vi "Check_Temps.vi"(8 "error in (no error)":errorcluster, 10 "Temperatures":sgl[][](array[numeric]), 11 "Alarm_Data In":T4) -> (0 "error out":errorcluster, 3 "Alarm_Data out":T4)   [LabVIEW 2019, in "Alarm_Manager.lvlib"]
uses:
  Alarm_Manager.lvlib
  Alarm_Data.ctl
  Message_Handler/typedef/Alarm_Panel.ctl
  Channel_Temperature_Threshold.ctl
  Open_Circuit.ctl
  Alarm.ctl
  Alarm_State_Enum.ctl
  Thermocouple.ctl
panel:
  out "Array":T1[](array[typedef])
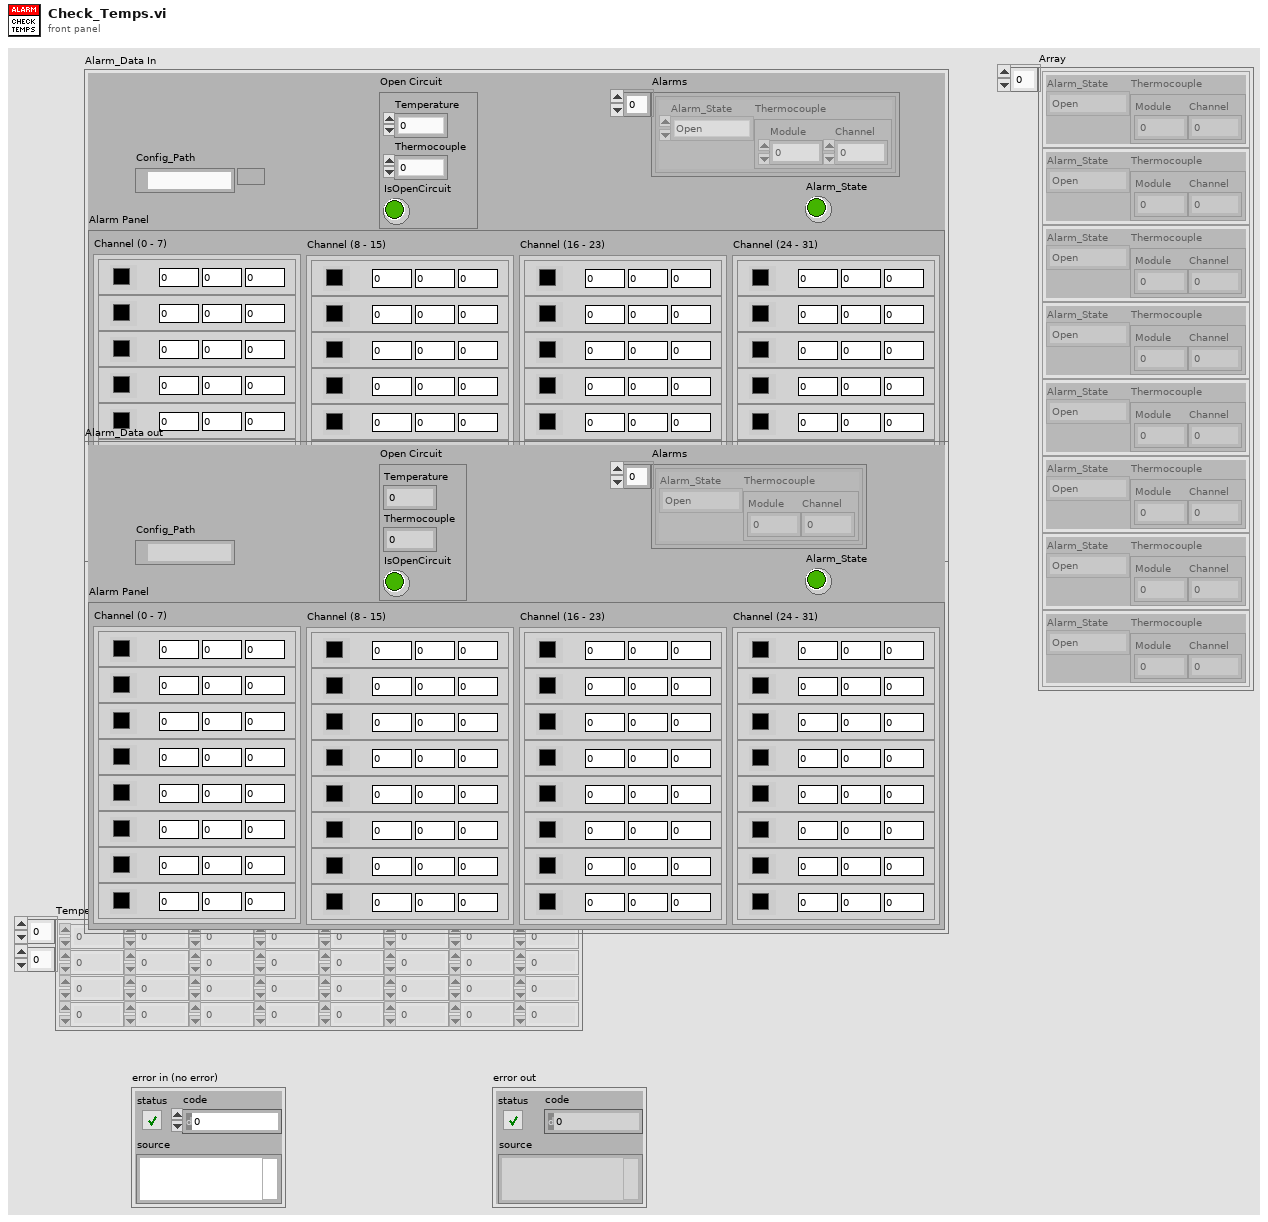
[diagram p1: front panel]
types:
  T1 = typedef "Alarm.ctl" = cluster{"Alarm_State":T2, "Thermocouple":T3}
  T2 = typedef "Alarm_State_Enum.ctl" = enum16{"Open", "Alarm", "None"}
  T3 = typedef "Thermocouple.ctl" = cluster{"Module":i32, "Channel":i32}
  T4 = typedef "Alarm_Data.ctl" = cluster{"Alarm Panel":T5, "Alarm_State":bool, "Config_Path":path, "Open Circuit":T7, "Alarms":T1[]}
  T5 = typedef "Alarm_Panel.ctl" = cluster{"Channel (0 - 7)":cluster{"Channel Temperature Thresholds":T6, "Channel Temperature Thresholds 2":T6, "Channel Temperature Thresholds 3":T6, "Channel Temperature Thresholds 4":T6, "Channel Temperature Thresholds 5":T6, "Channel Temperature Thresholds 6":T6, "Channel Temperature Thresholds 7":T6, "Channel Temperature Thresholds 8":T6}, "Channel (8 - 15)":cluster{"Channel Temperature Thresholds":T6, "Channel Temperature Thresholds 2":T6, "Channel Temperature Thresholds 3":T6, "Channel Temperature Thresholds 4":T6, "Channel Temperature Thresholds 5":T6, "Channel Temperature Thresholds 6":T6, "Channel Temperature Thresholds 7":T6, "Channel Temperature Thresholds 8":T6}, "Channel (16 - 23)":cluster{"Channel Temperature Thresholds":T6, "Channel Temperature Thresholds 2":T6, "Channel Temperature Thresholds 3":T6, "Channel Temperature Thresholds 4":T6, "Channel Temperature Thresholds 5":T6, "Channel Temperature Thresholds 6":T6, "Channel Temperature Thresholds 7":T6, "Channel Temperature Thresholds 8":T6}, "Channel (24 - 31)":cluster{"Channel Temperature Thresholds":T6, "Channel Temperature Thresholds 2":T6, "Channel Temperature Thresholds 3":T6, "Channel Temperature Thresholds 4":T6, "Channel Temperature Thresholds 5":T6, "Channel Temperature Thresholds 6":T6, "Channel Temperature Thresholds 7":T6, "Channel Temperature Thresholds 8":T6}}
  T6 = typedef "Channel_Temperature_Threshold.ctl" = cluster{"Min":i32, "Max":i32, "Alarm":i32, "Status":u32}
  T7 = typedef "Open_Circuit.ctl" = cluster{"Temperature":i32, "Thermocouple":i32, "IsOpenCircuit":bool}
  T8 = cluster{"Channel Temperature Thresholds":T6, "Channel Temperature Thresholds 2":T6, "Channel Temperature Thresholds 3":T6, "Channel Temperature Thresholds 4":T6, "Channel Temperature Thresholds 5":T6, "Channel Temperature Thresholds 6":T6, "Channel Temperature Thresholds 7":T6, "Channel Temperature Thresholds 8":T6}[]
  T9 = cluster{"[0]":T6, "[1]":T6, "[2]":T6, "[3]":T6, "[4]":T6, "[5]":T6, "[6]":T6, "[7]":T6}
  T10 = cluster{"[0]":cluster{"[0]":T6, "[1]":T6, "[2]":T6, "[3]":T6, "[4]":T6, "[5]":T6, "[6]":T6, "[7]":T6}, "[1]":cluster{"[0]":T6, "[1]":T6, "[2]":T6, "[3]":T6, "[4]":T6, "[5]":T6, "[6]":T6, "[7]":T6}, "[2]":cluster{"[0]":T6, "[1]":T6, "[2]":T6, "[3]":T6, "[4]":T6, "[5]":T6, "[6]":T6, "[7]":T6}, "[3]":cluster{"[0]":T6, "[1]":T6, "[2]":T6, "[3]":T6, "[4]":T6, "[5]":T6, "[6]":T6, "[7]":T6}}
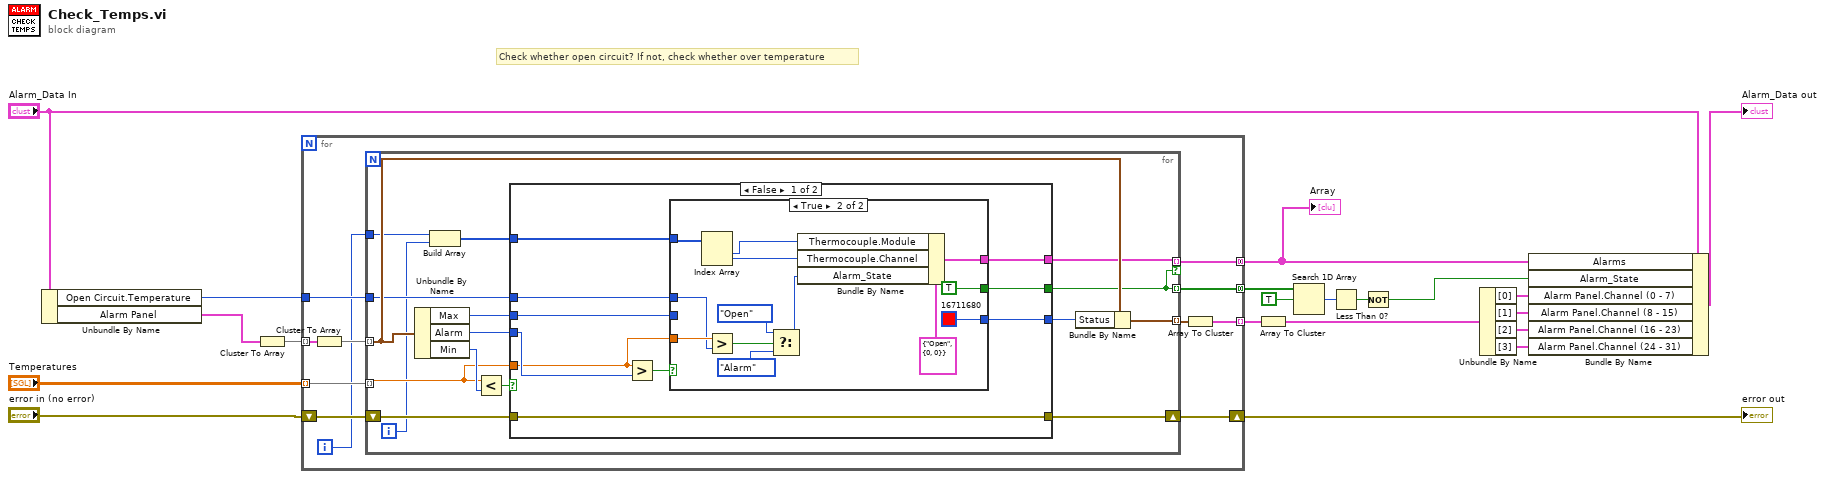
[diagram p0: block diagram]
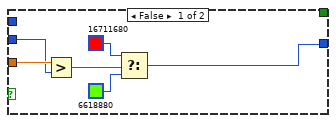
[diagram p2: hidden frame]
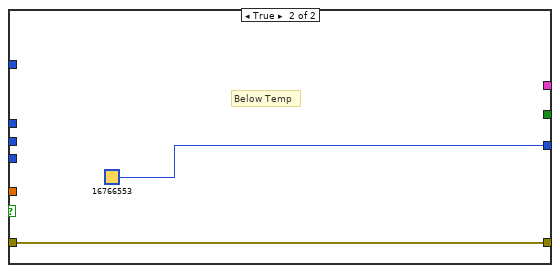
[diagram p3: hidden frame]
diagram:
  # "Check whether open circuit? If not, check whether over temperature"
  n1 = Unbundle By Name("Alarm_Data In") -> ("Open Circuit.Temperature"=w2:i32, "Alarm Panel"=w20:T5)
  n2 = Cluster To Array(cluster=w20) -> (array=w19:T8)
  n3 = for {
    tunnel: w19 -> [w31] mode=indexing
    tunnel: "Temperatures" -> [w29] mode=indexing
    shift-right: [w25] -> w16
    shift-left: "error in (no error)" -> [w28]
    tunnel: [w26] -> w15 mode=indexing
    tunnel: [w24] -> w7 mode=concatenating
    tunnel: w2 -> [w23]
    tunnel: [w21] -> w1 mode=concatenating
    i -> [w22]
    n4 = Cluster To Array(cluster=w31) -> (array=w30:T6[])
    n5 = for {
      tunnel: w30 -> [w42] mode=indexing
      tunnel: w29 -> [w45] mode=indexing
      shift-right: [w38] -> w25
      shift-left: w28 -> [w39]
      tunnel: [w40] -> w27 mode=indexing
      tunnel: [w32] -> w24 mode=indexing
      tunnel: w23 -> [w37]
      tunnel: w22 -> [w36]
      tunnel: [w33] -> w21 mode=indexing if=w32
      i -> [w35]
      n6 = Unbundle By Name(w42) -> ("Max"=w43:i32, "Alarm"=w44:i32, "Min"=w47:i32)
      n7 = Build Array(w36, w35) -> (w34:i32[])
      n8 = Less?(x=w45, y=w47) -> (x < y?=w46:bool)
      n9 = case shown="False" w46 {
        tunnel: w45 -> [w51 _]
        tunnel: w44 -> [w57 _]
        tunnel: w43 -> [w56 _]
        tunnel: [w55 u32 16766553] -> w41
        tunnel: w39 -> [w54 w77]
        tunnel: [w54 w77] -> w38
        tunnel: [w53 _] -> w32
        tunnel: w37 -> [w50 _]
        tunnel: w34 -> [w49 _]
        tunnel: [w48 _] -> w33
        frame False {
          n10 = Greater?(x=w51, y=w57) -> (0:w52:bool)
          n11 = case shown="True" w52 {
            tunnel: w51 -> [w63 w72]
            tunnel: w56 -> [w62 _]
            tunnel: [w58 u32 16711680] -> w55
            tunnel: [_ TRUE] -> w53
            tunnel: w50 -> [_ w71]
            tunnel: w49 -> [_ w67]
            tunnel: [_ w64] -> w48
            frame False {
              n12 = Greater?(x=w63, y=w62) -> (0:w60:bool)
              n13 = Select(t=u32 16711680, s=w60, f=u32 6618880) -> (s? t:f=w58:u32)
            }
            frame True {
              n14 = Index Array(array=w67) -> (element #1=w66:i32, element #2=w65:i32)  [unwired: 2 in]
              n15 = Greater?(x=w72, y=w71) -> (0:w70:bool)
              n16 = Select(t=Alarm_State_Enum."Open" ("Alarm_State"), s=w70, f=Alarm_State_Enum."Alarm" ("Alarm_State")) -> (s? t:f=w68:T2)
              n17 = Bundle By Name(cluster=T1 {"Alarm_State"=enum."Open", "Thermocouple"={"Module"=0, "Channel"=0}} ("Alarm"), "Thermocouple.Module"=w66, "Thermocouple.Channel"=w65, "Alarm_State"=w68) -> (w64:T1)
            }
          }
        }
        frame True {
          # "Below Temp"
        }
      }
      n18 = Bundle By Name(cluster=w42, "Status"=w41) -> (w40:T6)
    }
    n19 = Array To Cluster(array=w27) -> (cluster=w26:T9)
  }
  "error out" <- w16
  "Array" <- w1
  n20 = Array To Cluster(array=w15) -> (cluster=w14:T10)
  n21 = Search 1D Array(1D array=w7, element=TRUE) -> (index of element=w5:i32)  [unwired: 1 in]
  n22 = Less Than 0?(x=w5) -> (x < 0?=w4:bool)
  n23 = Not(x=w4) -> (.not. x?=w3:bool)
  n24 = Unbundle By Name(w14) -> ("[0]"=w11:T9, "[1]"=w10:T9, "[2]"=w9:T9, "[3]"=w8:T9)
  n25 = Bundle By Name(cluster="Alarm_Data In", "Alarms"=w1, "Alarm_State"=w3, "Alarm Panel.Channel (0 - 7)"=w11, "Alarm Panel.Channel (8 - 15)"=w10, "Alarm Panel.Channel (16 - 23)"=w9, "Alarm Panel.Channel (24 - 31)"=w8) -> (→"Alarm_Data out":T4)
